vi "getScreenBounds.vi"(0 "reference":refnum<class "Graphics.lvclass">, 5 "error in (no error)":errorcluster) -> (14 "reference out":refnum<class "Graphics.lvclass">, 15 "bounds":T1 {"height" format="%.2f"; "width" format="%.2f"; "y" format="%.2f"; "x" format="%.2f"}, 16 "ZoomChanged":bool, 19 "error out":errorcluster)   [LabVIEW 2012, in "Graphics.lvclass"]
doc: "Gets the bounds of the screen"
uses:
  <resource>/Framework/Providers/Open_GDS/UML/Graphics_class/Graphics.lvclass
  <resource>/Framework/Providers/Open_GDS/UML/General/Rectangle/Rectangle Rectangle2D.ctl
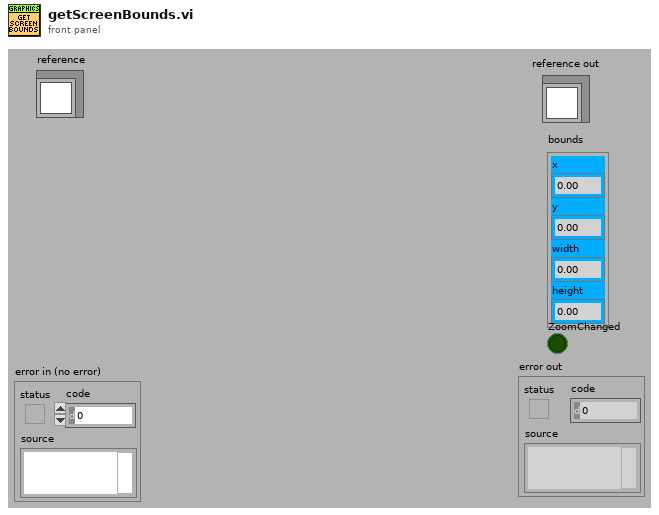
[diagram p1: front panel]
types:
  T1 = typedef "Rectangle Rectangle2D.ctl" = cluster{"x":dbl, "y":dbl, "width":dbl, "height":dbl}
  T2 = typedef "Graphics.lvclass/ObjectAttributes.ctl" = cluster{"drawColor":u32, "backgroundColor":u32, "font":T3, "fontType":T4, "picture":picture, "stroke":T5, "scaleX":dbl, "scaleY":dbl, "screenRef":refnum<vi>, "offsetX":dbl, "offsetY":dbl}
  T3 = typedef "Graphics.lvclass/FontType.ctl" = cluster{"Font Name:":string, "Size":i16, "Strikeout?":bool, "Italic?":bool, "Underline?":bool, "Outline?":bool, "Shadow?":bool, "Bold?":bool}
  T4 = typedef "Graphics.lvclass/LvFontType.ctl" = enum16{"User-specified Font", "Application Font", "System Font", "Dialog Font"}
  T5 = typedef "Graphics.lvclass/StrokeType.ctl" = enum16{"USE_DEFAULT", "SOLID", "DOTTED"}
  T6 = typedef "LVBoundsTypeDef.ctl" = cluster{"Width":u32, "Height":u32}
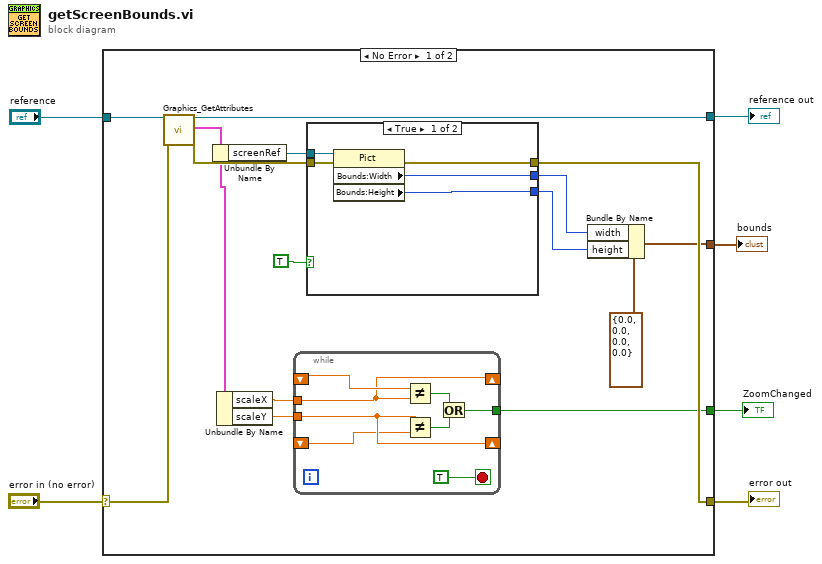
[diagram p0: block diagram]
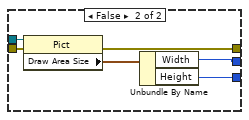
[diagram p2: hidden frame]
diagram:
  n1 = case shown="No Error" "error in (no error)" {
    selector: "error in (no error)" -> [w21 w41]
    tunnel: "reference" -> [w20 w42]
    tunnel: [w16 w41] -> w4
    tunnel: [w19 w42] -> w3
    tunnel: [w12 _] -> w2
    tunnel: [w8 _] -> w1
    frame No Error {
      n2 = call <resource>:"Graphics_GetAttributes.vi"("reference in"=w20, "error in (no error)"=w21) -> ("reference out"=w19:refnum<class "Graphics.lvclass">, "Data"=w7:T2, "error out"=w17:errorcluster)  [unwired: 1 in, 14 out]
      n3 = Unbundle By Name(w7) -> ("screenRef"=w18:refnum<vi>)
      n4 = Unbundle By Name(w7) -> ("scaleX"=w10:dbl, "scaleY"=w9:dbl)
      n5 = while {
        shift-right: [w28] -> _
        shift-left: _ -> [w29]
        shift-right: [w27] -> _
        shift-left: _ -> [w26]
        tunnel: w10 -> [w28]
        tunnel: w9 -> [w27]
        tunnel: [w22] -> w8
        stop <- TRUE stop-if-true
        n6 = Not Equal?(x=w29, y=w28) -> (x != y?=w24:bool)
        n7 = Not Equal?(x=w27, y=w26) -> (x != y?=w23:bool)
        n8 = Or(x=w24, y=w23) -> (x .or. y?=w22:bool)
      }
      n9 = case shown="True" TRUE ("Case Constant\n(See Context Help)") {
        tunnel: w18 -> [w34 w40]
        tunnel: w17 -> [w33 w39]
        tunnel: [w32 w38] -> w16
        tunnel: [w31 w36] -> w14
        tunnel: [w30 w35] -> w13
        frame True {
          n10 = property class="Pict"(reference=w34, error in=w33) -> (error out=w32:errorcluster, "Bounds:Width"=w31:u32, "Bounds:Height"=w30:u32)  [unwired: 1 out]
        }
        frame False {
          n11 = property class="Pict"(reference=w40, error in=w39) -> (error out=w38:errorcluster, "Draw Area Size"=w37:T6)  [unwired: 1 out]
          n12 = Unbundle By Name(w37) -> ("Width"=w36:u32, "Height"=w35:u32)
        }
      }
      n13 = Bundle By Name(cluster=T1 {"x"=0.0, "y"=0.0, "width"=0.0, "height"=0.0} ("bounds"), "width"=w14, "height"=w13) -> (w12:T1)
    }
    frame Error {
    }
  }
  "reference out" <- w3
  "error out" <- w4
  "bounds" <- w2
  "ZoomChanged" <- w1
